vi "Car Wash - Main.vi"() -> ()   [LabVIEW 2010]
doc: "Car Wash Main VI. Allows setup of multiple wash steps and sim of car position. Shows current step."
uses:
  Controls/Wash Options Cluster_TDef.ctl
  Controls/Car Wash Indicators Cluster_TDef.ctl
  Controls/Car Position Slider_TDef.ctl
  StateMachineStates 1.ctl
  Controls/Timer Actions ENUM_TDef.ctl
  Controls/Step Control Methods ENUM_TDef.ctl
panel:
  in  "Stop Program":bool
  in  "Car Position Slider":T1 scale=0.0..4.0
  out "Elapsed Time":dbl format="%.2g"
  out "Car Wash Indicators":T2
  out "Wash Entry":bool
  in  "Start":bool
  in  "Wash Options":T3
  # "Entry Console"
  # "Car Wash Display"
  # "Car Position Simulator"
  # "Underbody Wash\nBug Remover"
  # "Pre-Soak\nH-P Wash\nL-P Wax\nSpot Free Rinse"
  # "Tire Shine\nAir Dry"
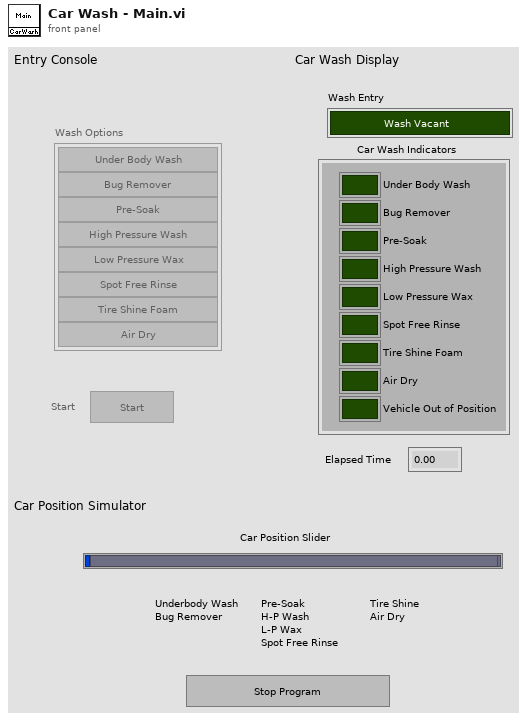
[diagram p1: front panel]
types:
  T1 = typedef "Car Position Slider_TDef.ctl" = u32
  T2 = typedef "Car Wash Indicators Cluster_TDef.ctl" = cluster{"Under Body Wash":bool, "Bug Remover":bool, "Pre-Soak":bool, "High Pressure Wash":bool, "Low Pressure Wax":bool, "Spot Free Rinse":bool, "Tire Shine Foam":bool, "Air Dry":bool, "Vehicle Out of Position":bool}
  T3 = typedef "Wash Options Cluster_TDef.ctl" = cluster{"Under Body Wash":bool, "Bug Remover":bool, "Pre-Soak":bool, "High Pressure Wash":bool, "Low Pressure Wax":bool, "Spot Free Rinse":bool, "Tire Shine Foam":bool, "Air Dry":bool}
  T4 = typedef "StateMachineStates 1.ctl" = enum16{"Initialize", "Wait for Start", "Run Position", "Reset", "Stop"}
  T5 = enum8{"Enabled", "Disabled", "Disabled and Grayed Out"}
  T6 = typedef "Times and Stations Cluster_TDef.ctl" = cluster{"Wash Times":dbl[], "Stations":T7[]}
  T7 = typedef "Stations ENUM_TDef.ctl" = enum16{"Station 1", "Station 2", "Station 3"}
  T8 = typedef "Timer Actions ENUM_TDef.ctl" = enum16{"Set Time", "Get Time", "Pause Time", "Resume Time"}
  T9 = typedef "Step Control Methods ENUM_TDef.ctl" = enum16{"Set Steps", "Get Current", "Goto Next Step"}
  T10 = typedef "Current Wash Step ENUM_TDef.ctl" = enum16{"Under Body Wash", "Bug Remover", "Pre-Soak", "High Pressure Wash", "Low Pressure Wax", "Spot Free Rinse", "Tire Shine Foam", "Air Dry"}
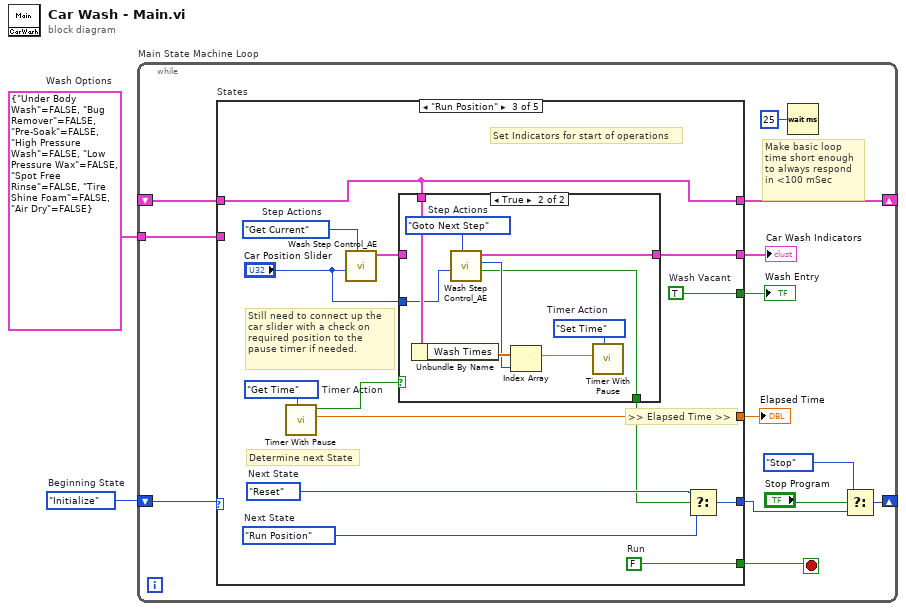
[diagram p0: block diagram]
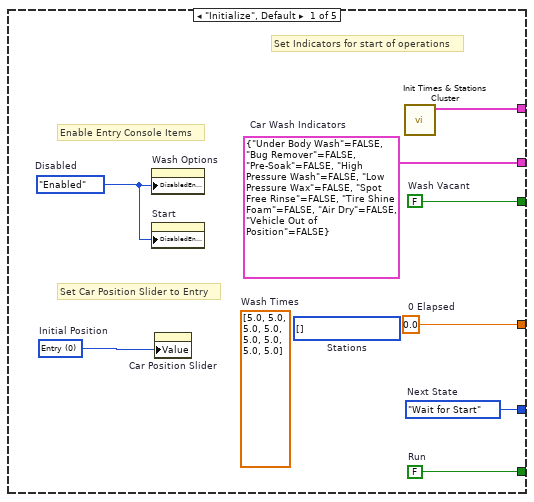
[diagram p2: hidden frame]
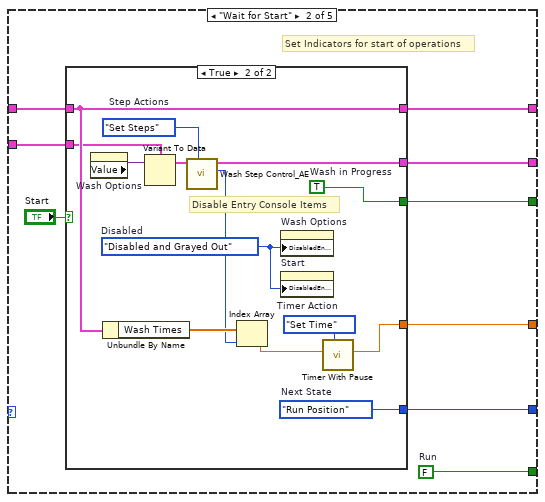
[diagram p3: hidden frame]
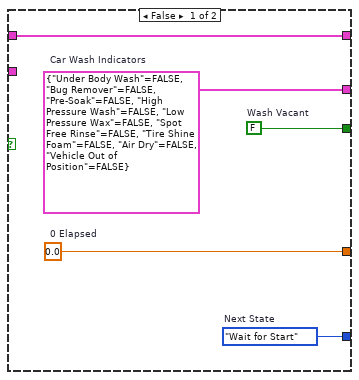
[diagram p4: hidden frame]
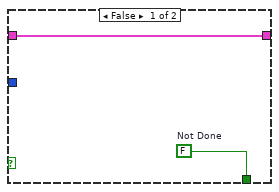
[diagram p5: hidden frame]
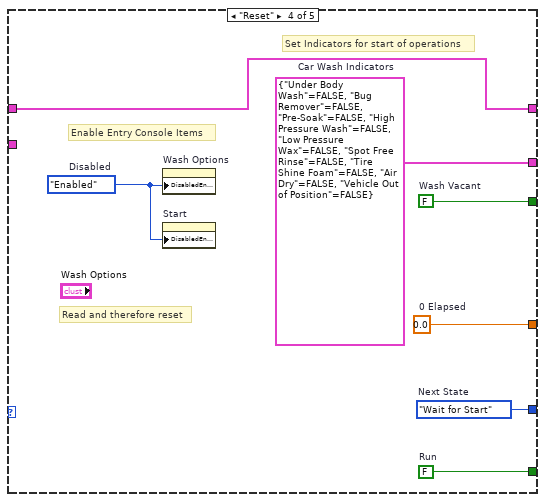
[diagram p6: hidden frame]
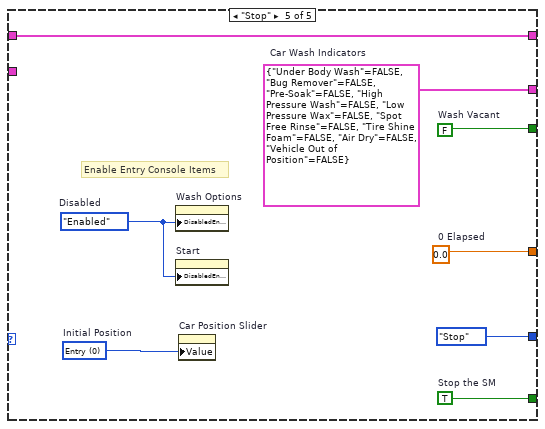
[diagram p7: hidden frame]
diagram:
  w1 = T3 {"Under Body Wash"=FALSE, "Bug Remover"=FALSE, "Pre-Soak"=FALSE, "High Pressure Wash"=FALSE, "Low Pressure Wax"=FALSE, "Spot Free Rinse"=FALSE, "Tire Shine Foam"=FALSE, "Air Dry"=FALSE}  # Wash Options
  w2 = StateMachineStates_1."Initialize"  # Beginning State
  n1 = while "Main State Machine Loop" {
    shift-right: [w11] -> _
    shift-left: w2 -> [w15]
    shift-right: [w5] -> _
    shift-left: _ -> [w7]
    tunnel: w1 -> [w3]
    stop <- w8 stop-if-true
    # "Make basic loop \ntime short enough\nto always respond\nin <100 mSec"
    n2 = case "States" shown="\"Run Position\"" w15 {
      tunnel: [w23 w25 w59 w83 StateMachineStates_1."Stop" ("Next State")] -> w12
      tunnel: [w21 w27 w62 w81 w89] -> w13
      tunnel: [w20 w32 w65 w80 w90] -> w8
      tunnel: w7 -> [_ w30 w54 w77 w88]
      tunnel: [w19 w28 w55 w79 w86] -> w6
      tunnel: [w16 w29 w54 w77 w88] -> w5
      tunnel: [w18 w26 w64 w78 w87] -> w4
      tunnel: w3 -> [_ w24 _ _ _]
      frame "Initialize", Default {
        (unwired) enum16{"Station 1", "Station 2", "Station 3"}[] [] items=["Station 1", "Station 2", "Station 3"]  # Stations
        (unwired) dbl[] [5.0, 5.0, 5.0, 5.0, 5.0, 5.0, 5.0, 5.0]  # Wash Times
        w17 = u32 0 items=["Entry", "Station 1", "Station 2", "Station 3", "Exit"]  # Initial Position
        w18 = FALSE  # Wash Vacant
        w19 = T2 {"Under Body Wash"=FALSE, "Bug Remover"=FALSE, "Pre-Soak"=FALSE, "High Pressure Wash"=FALSE, "Low Pressure Wax"=FALSE, "Spot Free Rinse"=FALSE, "Tire Shine Foam"=FALSE, "Air Dry"=FALSE, "Vehicle Out of Position"=FALSE}  # Car Wash Indicators
        w20 = FALSE  # Run
        w21 = 0.0  # 0 Elapsed
        w22 = T5."Enabled"  # Disabled
        w23 = StateMachineStates_1."Wait for Start"  # Next State
        # "Set Car Position Slider to Entry"
        # "Set Indicators for start of operations"
        # "Enable Entry Console Items"
        n3 = property on="Wash Options" class="Clust"("DisabledEnum"=w22) -> ()  [unwired: 2 in, 2 out]
        n4 = property on="Start" class="Bool"("DisabledEnum"=w22) -> ()  [unwired: 2 in, 2 out]
        n5 = property on="Car Position Slider" class="Slide (strict)"("Value"=w17) -> ()  [unwired: 2 in, 2 out]
        n6 = call "Init Times & Stations Cluster.vi"() -> ("Times and Stations"=w16:T6)  [unwired: 10 in, 1 out]
      }
      frame "Wait for Start" {
        w32 = FALSE  # Run
        # "Set Indicators for start of operations"
        n7 = case shown="True" "Start" {
          tunnel: w30 -> [w37 w46]
          tunnel: [w37 w46] -> w29
          tunnel: [w36 w49] -> w28
          tunnel: [w35 w47] -> w27
          tunnel: [w34 w42] -> w26
          tunnel: [w33 w41] -> w25
          tunnel: w24 -> [_ w38]
          frame False {
            w33 = StateMachineStates_1."Wait for Start"  # Next State
            w34 = FALSE  # Wash Vacant
            w35 = 0.0  # 0 Elapsed
            w36 = T2 {"Under Body Wash"=FALSE, "Bug Remover"=FALSE, "Pre-Soak"=FALSE, "High Pressure Wash"=FALSE, "Low Pressure Wax"=FALSE, "Spot Free Rinse"=FALSE, "Tire Shine Foam"=FALSE, "Air Dry"=FALSE, "Vehicle Out of Position"=FALSE}  # Car Wash Indicators
          }
          frame True {
            w41 = StateMachineStates_1."Run Position"  # Next State
            w42 = TRUE  # Wash in Progress
            w48 = Timer_Actions_ENUM_TDef."Set Time"  # Timer Action
            w50 = Step_Control_Methods_ENUM_TDef."Set Steps"  # Step Actions
            w51 = T5."Disabled and Grayed Out"  # Disabled
            # "Disable Entry Console Items"
            n8 = property on="Wash Options" class="Clust"() -> ("Value"=w40:variant)  [unwired: 2 in, 2 out]
            n9 = Unbundle By Name(w46) -> ("Wash Times"=w45:dbl[])
            n10 = Variant To Data(Variant=w40, type=w38) -> (data=w39:T3)  [unwired: 1 in, 1 out]
            n11 = call "Wash Step Control_AE.vi"("Step Actions"=w50, "Wash Options"=w39) -> ("Current Wash Step"=w44:T10, "Car Wash Indicators"=w49:T2)  [unwired: 6 in, 2 out]
            n12 = Index Array(array=w45, index=w44) -> (element=w43:dbl)
            n13 = property on="Wash Options" class="Clust"("DisabledEnum"=w51) -> ()  [unwired: 2 in, 2 out]
            n14 = property on="Start" class="Bool"("DisabledEnum"=w51) -> ()  [unwired: 2 in, 2 out]
            n15 = call "Timer With Pause.vi"("Timer Action"=w48, "Target Time"=w43) -> ("Elapsed Time"=w47:dbl)  [unwired: 6 in, 3 out]
          }
        }
      }
      frame "Run Position" {
        w60 = StateMachineStates_1."Run Position"  # Next State
        w61 = Step_Control_Methods_ENUM_TDef."Get Current"  # Step Actions
        w63 = Timer_Actions_ENUM_TDef."Get Time"  # Timer Action
        w64 = TRUE  # Wash Vacant
        w65 = FALSE  # Run
        w58 = StateMachineStates_1."Reset"  # Next State
        # "Still need to connect up the\ncar slider with a check on\nrequired position to the\npause timer if needed."
        # "Determine next State"
        # ">> Elapsed Time >>"
        # "Set Indicators for start of operations"
        n16 = call "Timer With Pause.vi"("Timer Action"=w63) -> ("Elapsed Time"=w62:dbl, "Done?"=w56:bool)  [unwired: 7 in, 2 out]
        n17 = call "Wash Step Control_AE.vi"("Step Actions"=w61, "Car Position Slider"="Car Position Slider") -> ("Car Wash Indicators"=w57:T2)  [unwired: 6 in, 3 out]
        n18 = case shown="True" w56 {
          tunnel: w57 -> [w67 _]
          tunnel: [w67 w75] -> w55
          tunnel: w54 -> [_ w73]
          tunnel: "Car Position Slider" -> [_ w69]
          tunnel: [w66 w68] -> w52
          frame False {
            w66 = FALSE  # Not Done
          }
          frame True {
            w74 = Timer_Actions_ENUM_TDef."Set Time"  # Timer Action
            w76 = Step_Control_Methods_ENUM_TDef."Goto Next Step"  # Step Actions
            n19 = Unbundle By Name(w73) -> ("Wash Times"=w72:dbl[])
            n20 = call "Wash Step Control_AE.vi"("Step Actions"=w76, "Car Position Slider"=w69) -> ("Done with Washing?"=w68:bool, "Current Wash Step"=w71:T10, "Car Wash Indicators"=w75:T2)  [unwired: 6 in, 1 out]
            n21 = Index Array(array=w72, index=w71) -> (element=w70:dbl)
            n22 = call "Timer With Pause.vi"("Timer Action"=w74, "Target Time"=w70) -> ()  [unwired: 6 in, 4 out]
          }
        }
        n23 = Select(t=w58, s=w52, f=w60) -> (s? t:f=w59:T4)
      }
      frame "Reset" {
        w78 = FALSE  # Wash Vacant
        w79 = T2 {"Under Body Wash"=FALSE, "Bug Remover"=FALSE, "Pre-Soak"=FALSE, "High Pressure Wash"=FALSE, "Low Pressure Wax"=FALSE, "Spot Free Rinse"=FALSE, "Tire Shine Foam"=FALSE, "Air Dry"=FALSE, "Vehicle Out of Position"=FALSE}  # Car Wash Indicators
        w80 = FALSE  # Run
        w81 = 0.0  # 0 Elapsed
        w82 = T5."Enabled"  # Disabled
        w83 = StateMachineStates_1."Wait for Start"  # Next State
        # "Read and therefore reset"
        # "Set Indicators for start of operations"
        # "Enable Entry Console Items"
        n24 = property on="Wash Options" class="Clust"("DisabledEnum"=w82) -> ()  [unwired: 2 in, 2 out]
        n25 = property on="Start" class="Bool"("DisabledEnum"=w82) -> ()  [unwired: 2 in, 2 out]
      }
      frame "Stop" {
        w84 = u32 0 items=["Entry", "Station 1", "Station 2", "Station 3", "Exit"]  # Initial Position
        w85 = T5."Enabled"  # Disabled
        w86 = T2 {"Under Body Wash"=FALSE, "Bug Remover"=FALSE, "Pre-Soak"=FALSE, "High Pressure Wash"=FALSE, "Low Pressure Wax"=FALSE, "Spot Free Rinse"=FALSE, "Tire Shine Foam"=FALSE, "Air Dry"=FALSE, "Vehicle Out of Position"=FALSE}  # Car Wash Indicators
        w87 = FALSE  # Wash Vacant
        w89 = 0.0  # 0 Elapsed
        w90 = TRUE  # Stop the SM
        # "Enable Entry Console Items"
        n26 = property on="Wash Options" class="Clust"("DisabledEnum"=w85) -> ()  [unwired: 2 in, 2 out]
        n27 = property on="Start" class="Bool"("DisabledEnum"=w85) -> ()  [unwired: 2 in, 2 out]
        n28 = property on="Car Position Slider" class="Slide (strict)"("Value"=w84) -> ()  [unwired: 2 in, 2 out]
      }
    }
    "Elapsed Time" <- w13
    "Car Wash Indicators" <- w6
    "Wash Entry" <- w4
    n29 = Wait (ms)(milliseconds to wait=u32 25) -> ()  [unwired: 1 out]
    n30 = Select(t=StateMachineStates_1."Stop" ("States"), s="Stop Program", f=w12) -> (s? t:f=w11:T4)
  }
